vi "Picture.vi"(0 "path to BMP file":path, 1 "XML File Path":path) -> ()   [LabVIEW 2010]
uses:
  <vilib>/xml/NI_XML.lvlib
  C:/Program Files (x86)/National Instruments/LabVIEW 2010/resource/objmgr/DOMUserDefRef.rc
panel:
  in  "Out":refnum<vi>
  in  "In":refnum<vi>
  out "Boolean":bool caption="out[0]"
  in  "XML File Path memory":path
  out "Boolean 3":bool caption="in[1]"
  out "Boolean 2":bool caption="in[0]"
  out "?":picture
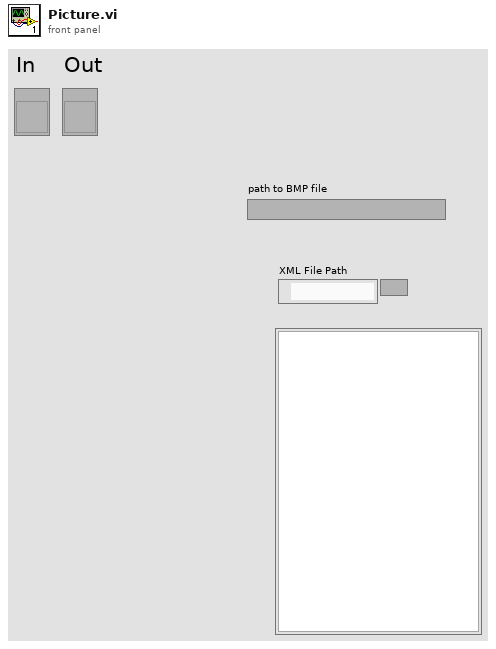
[diagram p1: front panel]
types:
  T1 = typedef "imagedata.ctl" = cluster{"image type":i32, "image depth":i32, "image":u8[], "mask":u8[], "colors":u32[], "Rectangle":cluster{"left":i16, "top":i16, "right":i16, "bottom":i16}}
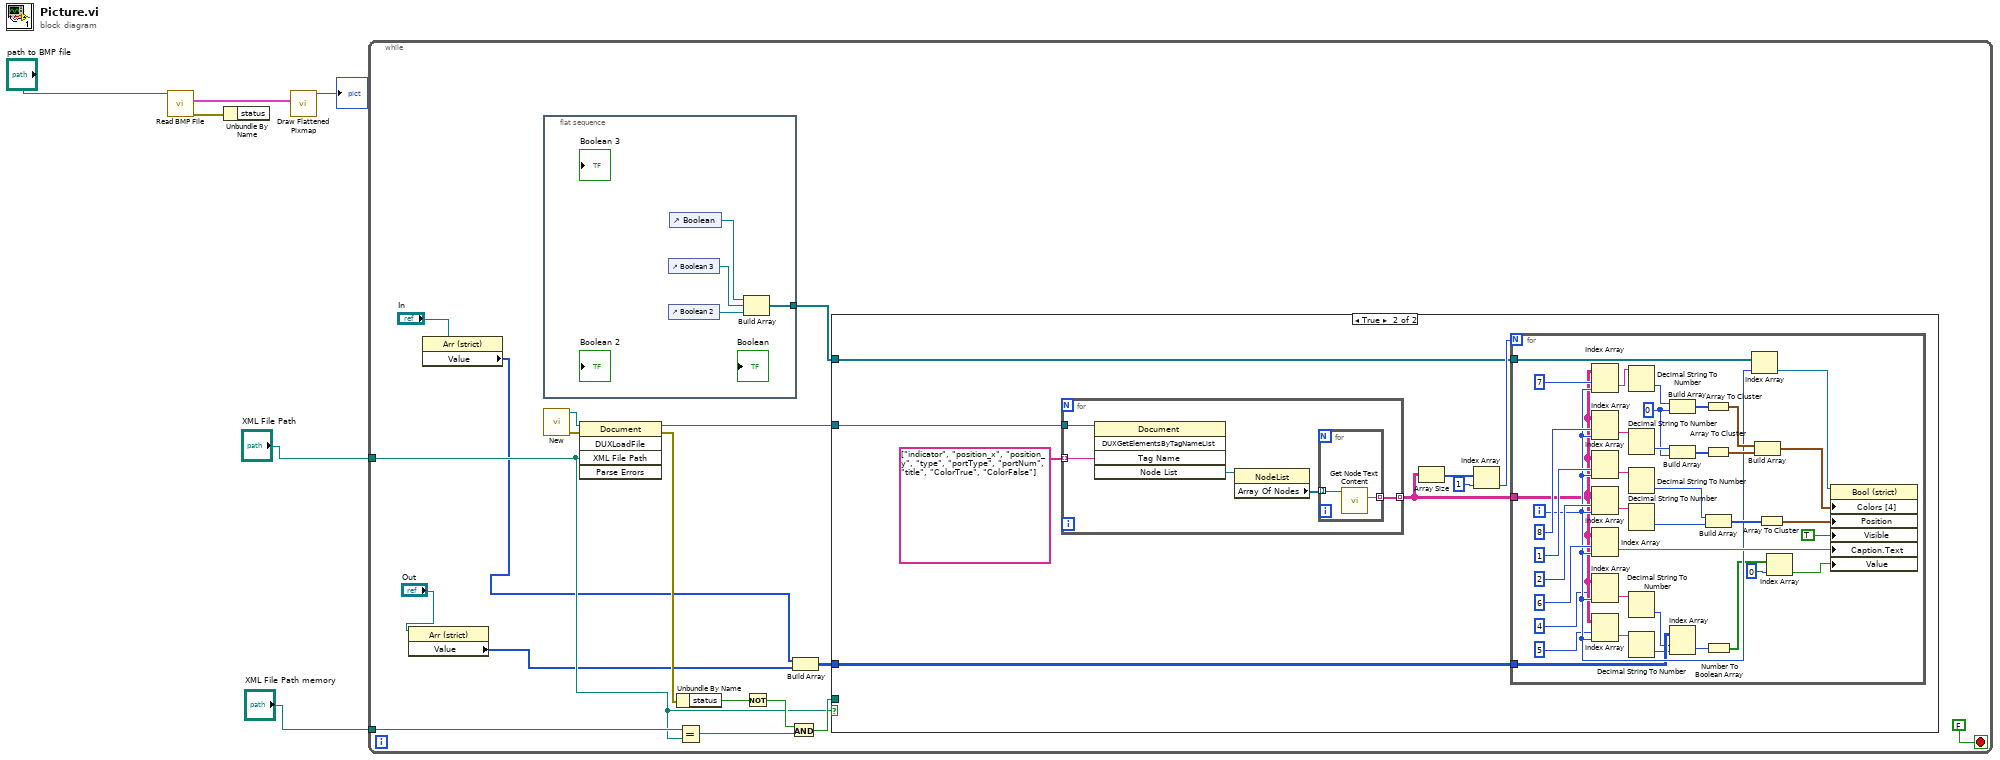
[diagram p0: block diagram]
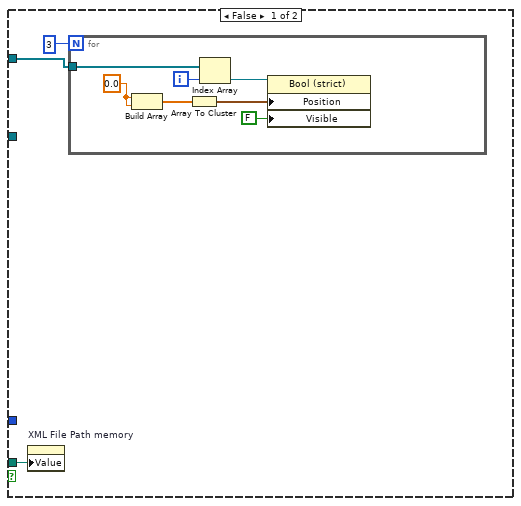
[diagram p2: hidden frame]
diagram:
  n1 = call <vilib>:"Read BMP File.vi"("path to BMP file"="path to BMP file") -> ("error out"=w4:errorcluster, "image data"=w3:T1)  [unwired: 8 in, 1 out]
  n2 = Unbundle By Name(w4) -> ()  [unwired: 1 out]
  n3 = call <vilib>:"Draw Flattened Pixmap.vi"("image data"=w3) -> ("new picture"=→"?":picture)  [unwired: 8 in]
  n4 = while {
    tunnel: "XML File Path memory" -> [w12]
    tunnel: "XML File Path" -> [w11]
    stop <- FALSE stop-if-true
    n5 = property class="Arr (strict)"(reference="Out") -> ("Value"=w7:i8[])  [unwired: 1 in, 2 out]
    n6 = property class="Arr (strict)"(reference="In") -> ("Value"=w9:i8[])  [unwired: 1 in, 2 out]
    n7 = flat-sequence {
      tunnel: [w25] -> w22
      frame #0 {
        n8 = control-ref of="Boolean 3"() -> (w26:refnum<vi>)
        n9 = control-ref of="Boolean 2"() -> (w24:refnum<vi>)
        n10 = control-ref of="Boolean"() -> (w27:refnum<vi>)
        n11 = Build Array(w27, w26, w24) -> (w25:refnum<vi>[])
      }
    }
    n12 = call <vilib>:"New.vi"() -> ("error out"=w21:errorcluster, "DOM document out"=w20:refnum<k20>)  [unwired: 8 in]
    n13 = invoke class="Document" method="DUXLoadFile"(reference=w20, error in=w21, "XML File Path"=w11) -> (reference out=w19:refnum<k20>, error out=w17:errorcluster)  [unwired: 2 in, 3 out]
    n14 = Unbundle By Name(w17) -> ("status"=w15:bool)
    n15 = Equal?(x=w12, y=w11) -> (x = y?=w18:bool)
    n16 = Not(x=w15) -> (.not. x?=w14:bool)
    n17 = And(x=w14, y=w18) -> (x .and. y?=w16:bool)
    n18 = Build Array(w9, w7) -> (w13:i8[][])
    n19 = case shown="True" w16 {
      tunnel: w11 -> [w29 _]
      tunnel: w22 -> [w28 w40]
      tunnel: w19 -> [_ w39]
      tunnel: w13 -> [_ w38]
      frame False {
        n20 = property on="XML File Path memory" class="Path"("Value"=w29) -> ()  [unwired: 2 in, 2 out]
        n21 = for {
          N: 3 -> [_]
          tunnel: w28 -> [w32]
          i -> [w31]
          w34 = 0.0 ("element")
          n22 = Build Array(w34, w34) -> (w37:dbl[])
          n23 = Array To Cluster(array=w37) -> (cluster=w35:cluster{"[0]":dbl, "[1]":dbl})
          n24 = Index Array(array=w32, index=w31) -> (element=w33:refnum<vi>)
          n25 = property on="Property Node" class="Bool (strict)"(reference=w33, "Position"=w35, "Visible"=FALSE) -> ()  [unwired: 1 in, 2 out]
        }
      }
      frame True {
        n26 = for {
          tunnel: string[] ["indicator", "position_x", "position_y", "type", "portType", "portNum", "title", "ColorTrue", "ColorFalse"] -> [w48] mode=indexing
          tunnel: [w47] -> w44 mode=indexing
          tunnel: w39 -> [w46]
          n27 = invoke class="Document" method="DUXGetElementsByTagNameList"(reference=w46, "Tag Name"=w48) -> ("Node List"=w50:refnum<k20>)  [unwired: 3 in, 4 out]
          n28 = property class="NodeList"(reference=w50) -> ("Array Of Nodes"=w49:refnum<k20>[])  [unwired: 1 in, 2 out]
          n29 = for {
            tunnel: w49 -> [w52] mode=indexing
            tunnel: [w51] -> w47 mode=indexing
            n30 = call <vilib>:"Get Node Text Content.vi"("node in"=w52) -> ("node text"=w51:string)  [unwired: 8 in, 2 out]
          }
        }
        n31 = Array Size(array=w44) -> (size(s)=w43:i32[])
        n32 = Index Array(array=w43, index=1) -> (element=w42:i32)
        n33 = for {
          N: w42 -> [_]
          tunnel: w44 -> [w64]
          tunnel: w40 -> [w66]
          tunnel: w38 -> [w61]
          i -> [w65]
          w68 = 0 ("element")
          n34 = Index Array(array=w64, index (row)=7 ("disabled index (row)"), index (col)=w65) -> (element=w75:string)
          n35 = Index Array(array=w64, index (row)=8 ("disabled index (row)"), index (col)=w65) -> (element=w76:string)
          n36 = Index Array(array=w64, index (row)=1 ("disabled index (row)"), index (col)=w65) -> (element=w87:string)
          n37 = Index Array(array=w64, index (row)=2 ("disabled index (row)"), index (col)=w65) -> (element=w88:string)
          n38 = Index Array(array=w64, index (row)=6 ("disabled index (row)"), index (col)=w65) -> (element=w80:string)
          n39 = Index Array(array=w64, index (row)=4, index (col)=w65) -> (element=w59:string)
          n40 = Index Array(array=w64, index (row)=5, index (col)=w65) -> (element=w60:string)
          n41 = Decimal String To Number(string=w75) -> (number=w77:i32)  [unwired: 2 in, 1 out]
          n42 = Decimal String To Number(string=w76) -> (number=w69:i32)  [unwired: 2 in, 1 out]
          n43 = Decimal String To Number(string=w87) -> (number=w86:i32)  [unwired: 2 in, 1 out]
          n44 = Decimal String To Number(string=w88) -> (number=w85:i32)  [unwired: 2 in, 1 out]
          n45 = Decimal String To Number(string=w59) -> (number=w54:i32)  [unwired: 2 in, 1 out]
          n46 = Decimal String To Number(string=w60) -> (number=w53:i32)  [unwired: 2 in, 1 out]
          n47 = Build Array(w77, w68) -> (w73:i32[])
          n48 = Build Array(w69, w68) -> (w72:i32[])
          n49 = Index Array(array=w61, index (row)=w54, index (col)=w53) -> (element=w55:i8)
          n50 = Array To Cluster(array=w73) -> (cluster=w70:cluster{"[0]":i32, "[1]":i32})
          n51 = Array To Cluster(array=w72) -> (cluster=w71:cluster{"[0]":i32, "[1]":i32})
          n52 = Build Array(w86, w85) -> (w84:i32[])
          n53 = Number To Boolean Array(number=w55) -> (Boolean array=w56:bool[])
          n54 = Index Array(array=w66, index=w65) -> (element=w67:refnum<vi>)
          n55 = Build Array(w70, w71) -> (w74:cluster{"[0]":i32, "[1]":i32}[])
          n56 = Array To Cluster(array=w84) -> (cluster=w82:cluster{"[0]":i32, "[1]":i32})
          n57 = Index Array(array=w56, index=0) -> (element=w57:bool)
          n58 = property on="Property Node" class="Bool (strict)"(reference=w67, "Colors [4]"=w74, "Position"=w82, "Visible"=TRUE, "Caption.Text"=w80, "Value"=w57) -> ()  [unwired: 1 in, 2 out]
        }
      }
    }
  }
